vi "Stop Acquisition.vi"(8 "error in (no error)":errorcluster, 11 "Acquisition in":refnum<class "Acquisition.lvclass">) -> (0 "error out":errorcluster)   [LabVIEW 2018, in "Acquisition.lvlib" / "Acquisition.lvclass"]
doc: "Stops the acquisition.\n_____\nBased on Delacor QMH Project Template 4.2.0.62."
uses:
  Acquisition.lvclass
  Acquisition.lvclass/Acquisition.ctl
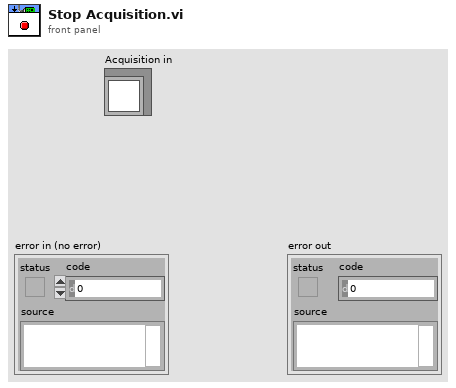
[diagram p1: front panel]
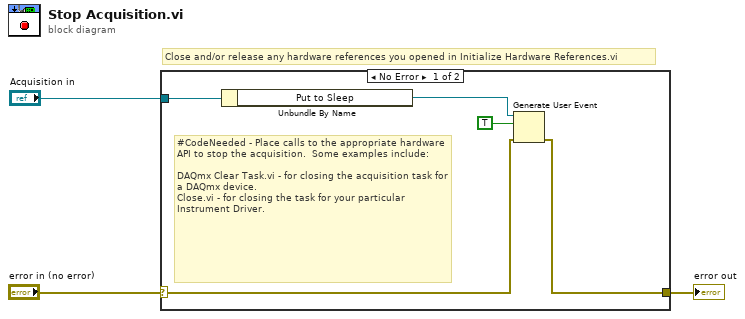
[diagram p0: block diagram]
diagram:
  # "Close and/or release any hardware references you opened in Initialize Hardware References.vi"
  n1 = case shown="No Error" "error in (no error)" {
    selector: "error in (no error)" -> [w6 w9]
    tunnel: [w5 w9] -> w2
    tunnel: "Acquisition in" -> [w8 _]
    frame No Error {
      # "#CodeNeeded - Place calls to the appropriate hardware API to stop the acquisition.  Some examples include:\n\nDAQmx Clear Task.vi - for closing the acquisition task for a DAQmx device.\nClose.vi - for closing the task for your particular Instrument Driver."
      n2 = Unbundle By Name(w8) -> ("Put to Sleep"=w7:refnum<user-event>)
      n3 = Generate User Event(user event=w7, event data cluster=TRUE ("event data"), error in=w6) -> (error out=w5:errorcluster)  [unwired: 1 in, 1 out]
    }
    frame Error {
    }
  }
  "error out" <- w2
